vi "SafeMovementToPosition.vi"(10 "Target position":dbl, 11 "Connection Cluster in":T1) -> (3 "Connection Cluster out":T1)   [LabVIEW 2013]
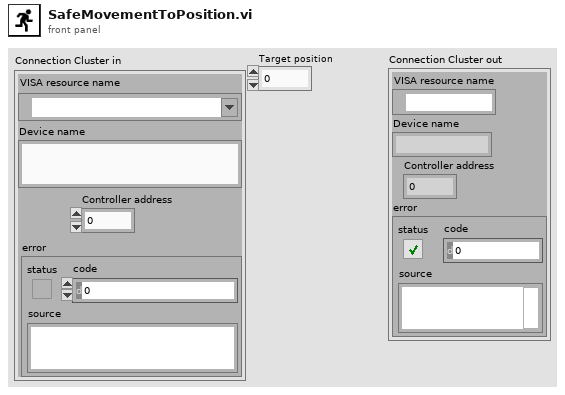
[diagram p1: front panel]
types:
  T1 = cluster{"VISA resource name":refnum<visa-resource-name>, "Device name":string, "Controller address":i32, "error":errorcluster}
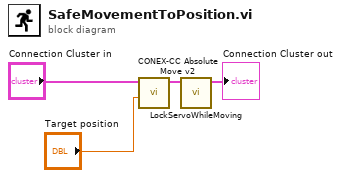
[diagram p0: block diagram]
diagram:
  n1 = call <userlib>:"CONEX-CC Absolute Move v2.vi"("Target position"="Target position", "Connection Cluster in"="Connection Cluster in") -> ("Connection Cluster out"=w1:T1)  [unwired: 7 in]
  n2 = call "LockServoWhileMoving.vi"("Connection Cluster in"=w1) -> ("Connection Cluster out 2"=→"Connection Cluster out":T1)  [unwired: 10 in]
